vi "Create from string.vi"(8 "error in (no error)":errorcluster, 11 "address":string) -> (0 "error out":errorcluster, 3 "Hostname Network Address out":refnum<class "Generic Network Address.lvclass">)   [LabVIEW 2020, in "NI_WFCN.lvlib" / "Hostname Network Address.lvclass"]
doc: "Constructs a Hostname Network Address object representing the specified hostname."
uses:
  <vilib>/net/WFCN/Addressing/Hostname Network Address/Hostname Network Address.lvclass
  <vilib>/net/WFCN/Addressing/Generic Network Address/Generic Network Address.lvclass
  <vilib>/net/WFCN/Addressing/Generic Network Address/Generic Network Address.lvclass/Generic Network Address.ctl
  e:/builds/penguin/labview/branches/2020/dev/dist/vi.lib/net/WFCN/Addressing/Generic Network Address/Generic Network Address.lvclass
  <vilib>/net/WFCN/Addressing/mDNS Hostname Network Address/mDNS Hostname Network Address.lvclass
  e:/builds/penguin/labview/branches/2020/dev/dist/vi.lib/net/WFCN/Addressing/Hostname Network Address/Hostname Network Address.lvclass
  <vilib>/net/WFCN/Addressing/Hostname Network Address/Hostname Network Address.lvclass/Hostname Network Address.ctl
  <vilib>/net/WFCN/NI_WFCN.lvlib
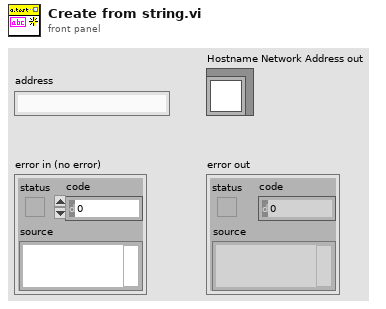
[diagram p1: front panel]
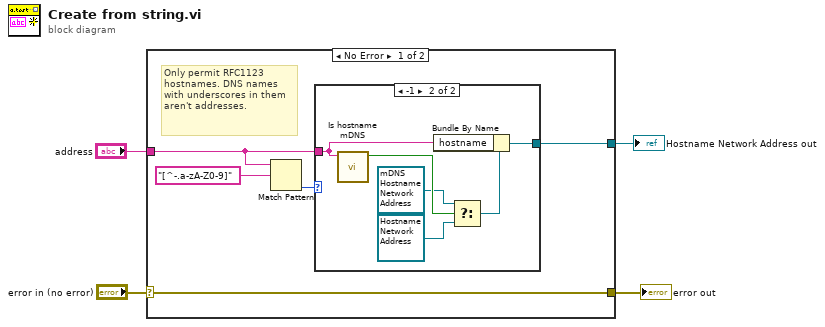
[diagram p0: block diagram]
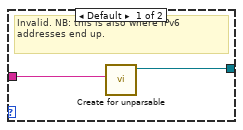
[diagram p2: hidden frame]
diagram:
  n1 = case shown="No Error" "error in (no error)" {
    selector: "error in (no error)" -> [w6 w18]
    tunnel: [w9 _] -> w4
    tunnel: "address" -> [w8 _]
    tunnel: [w6 w18] -> w2
    frame No Error {
      # "Only permit RFC1123 hostnames. DNS names with underscores in them aren't addresses."
      n2 = Match Pattern(string=w8, regular expression="[^-.a-zA-Z0-9]") -> (offset past match=w5:i32)  [unwired: 1 in, 3 out]
      n3 = case shown="-1" w5 {
        tunnel: w8 -> [w11 w12]
        tunnel: [w10 w13] -> w9
        frame Default {
          # "Invalid. NB: this is also where IPv6 addresses end up."
          n4 = call <vilib>:"Create for unparsable.vi"("hostname"=w11) -> ("Generic Network Address out"=w10:refnum<class "Generic Network Address.lvclass">)  [unwired: 10 in]
        }
        frame -1 {
          n5 = call <vilib>:"Is hostname mDNS.vi"("address"=w12) -> ("mDNS?"=w17:bool)  [unwired: 10 in]
          n6 = Select(t=refnum<class "mDNS Hostname Network Address.lvclass"> refnum ("mDNS Hostname Network Address.lvclass"), s=w17, f=refnum<class "Hostname Network Address.lvclass"> refnum ("Hostname Network Address in")) -> (s? t:f=w14:refnum<class "Hostname Network Address.lvclass">)
          n7 = Bundle By Name(cluster=w14, "hostname"=w12) -> (w13:refnum<class "Hostname Network Address.lvclass">)
        }
      }
    }
    frame Error {
    }
  }
  "error out" <- w2
  "Hostname Network Address out" <- w4
